vi "CT-Init Jitter.vi"(0 "Num Components":i32, 5 "Min F0 (Hz)":dbl, 7 "% jitter":dbl) -> (4 "frequency multipliers":dbl[](array[numeric]))   [LabVIEW 2015]
uses:
  Utility VIs/Math VIs/LinSpace (x0-dx-npts).vi
  <vilib>/Analysis/NI_AALBase.lvlib
  <vilib>/Analysis/NI_AALPro.lvlib
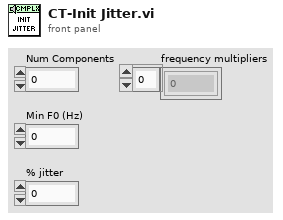
[diagram p1: front panel]
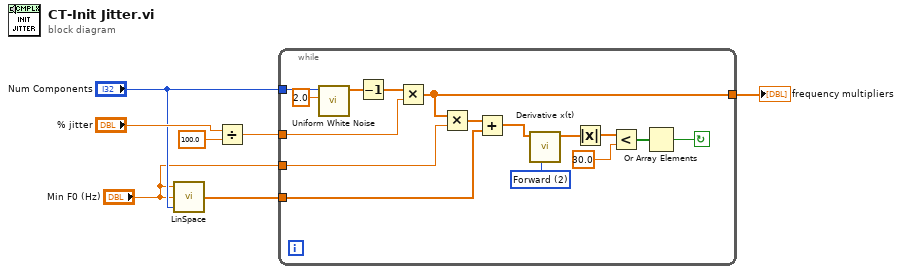
[diagram p0: block diagram]
diagram:
  n1 = call-poly "LinSpace.vi"("npts"="Num Components", "dx"="Min F0 (Hz)", "x0"="Min F0 (Hz)") -> ("Array"=w2:dbl[])  [unwired: 1 in, 1 out]
  n2 = Divide(x="% jitter", y=100.0) -> (x/y=w6:dbl)
  n3 = while {
    tunnel: w6 -> [w20]
    tunnel: [w19] -> w4
    tunnel: "Num Components" -> [w18]
    tunnel: w2 -> [w9]
    tunnel: "Min F0 (Hz)" -> [w8]
    stop <- w11 continue-if-true
    w17 = u16 2 items=["2nd Order Central", "4th Order Central", "Forward", "Backward"] ("method")
    n4 = call <vilib>:"Uniform White Noise.vi"("amplitude"=2.0, "samples"=w18) -> ("uniform white noise"=w22:dbl[])  [unwired: 8 in, 1 out]
    n5 = Decrement(x=w22) -> (x-1=w21:dbl[])
    n6 = Multiply(x=w21, y=w20) -> (x*y=w19:dbl[])
    n7 = Multiply(x=w19, y=w8) -> (x*y=w16:dbl[])
    n8 = Add(x=w16, y=w9) -> (x+y=w10:dbl[])
    n9 = call <vilib>:"Derivative x(t).vi"("method"=w17, "X"=w10) -> ("dX/dt"=w15:dbl[])  [unwired: 8 in, 1 out]
    n10 = Absolute Value(x=w15) -> (abs(x)=w14:dbl[])
    n11 = Less?(x=w14, y=30.0) -> (x < y?=w12:bool[])
    n12 = Or Array Elements(Boolean array=w12) -> (logical OR=w11:bool)
  }
  "frequency multipliers" <- w4
